vi "Coerce Panel Bounds to Fit Minimum Size.vi"(10 "minimum panel size":T2, 11 "FP panel bounds in":T1) -> (3 "FP panel bounds out":T1)   [LabVIEW 2010, in "NI_SE_Front Panel Layout.lvlib"]
uses:
  NI_SE_Front Panel Layout.lvlib
  <vilib>/Utility/miscctls.llb/LVPointTypeDef.ctl
  <vilib>/Utility/miscctls.llb/LVRectTypeDef.ctl
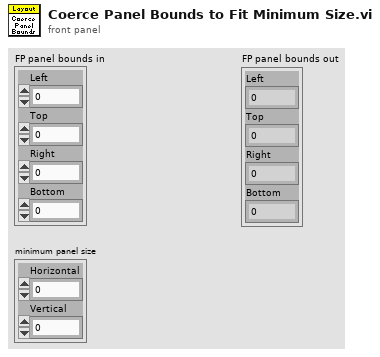
[diagram p1: front panel]
types:
  T1 = typedef "LVRectTypeDef.ctl" = cluster{"Left":i16, "Top":i16, "Right":i16, "Bottom":i16}
  T2 = typedef "LVPointTypeDef.ctl" = cluster{"Horizontal":i16, "Vertical":i16}
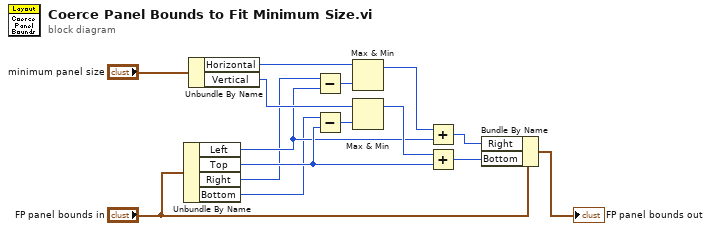
[diagram p0: block diagram]
diagram:
  n1 = Unbundle By Name("FP panel bounds in") -> ("Left"=w9:i16, "Top"=w13:i16, "Right"=w4:i16, "Bottom"=w5:i16)
  n2 = Unbundle By Name("minimum panel size") -> ("Horizontal"=w6:i16, "Vertical"=w10:i16)
  n3 = Subtract(x=w4, y=w9) -> (x-y=w7:i16)
  n4 = Subtract(x=w5, y=w13) -> (x-y=w11:i16)
  n5 = Max & Min(x=w6, y=w7) -> (max(x,y)=w8:i16)  [unwired: 1 out]
  n6 = Max & Min(x=w10, y=w11) -> (max(x,y)=w12:i16)  [unwired: 1 out]
  n7 = Add(x=w8, y=w9) -> (x+y=w14:i16)
  n8 = Add(x=w12, y=w13) -> (x+y=w15:i16)
  n9 = Bundle By Name(cluster="FP panel bounds in", "Right"=w14, "Bottom"=w15) -> (→"FP panel bounds out":T1)
